vi "Import Data Sharing Framework with UDP Component.vi"() -> (3 "Output System Definition File":path)   [LabVIEW 2020, in "Data Sharing Framework Scripting Examples.lvlib"]
uses:
  Data Sharing Framework Scripting Examples.lvlib
  NationalInstruments.VeriStand.SystemDefinitionAPI
  <vilib>/addons/VeriStand Custom Device Scripting APIs/Data Sharing Framework/Data Sharing Framework Custom Device Scripting.lvlib
panel:
  in  "Launch Data Viewer":bool=TRUE
  in  "Data Server Frequency":dbl(ring)=10.0 items=["0.5 Hz"=0.5, "1.0 Hz"=1.0, "2.0 Hz"=2.0, "2.5 Hz"=2.5, "4.0 Hz"=4.0, "5.0 Hz"=5.0, "8.0 Hz"=8.0, "10.0 Hz"=10.0, "12.5 Hz"=12.5, "20.0 Hz"=20.0, "25.0 Hz"=25.0, "40.0 Hz"=40.0, "50.0 Hz"=50.0, "100.0 Hz"=100.0]
  in  "Enable Data Server":bool=TRUE
  # "Overview: Demonstrates using the Data Sharing Framework scripting API to import a UDP plugin for data communication between VeriStand and LabVIEW. \n\nInstructions:\n1. Specify data server parameters. \n2. You may specify configuration and system definition files on the Block Diagram.\n3. Run this VI to import the DSF configuration, save the system definition.\n4. From VeriStand, run the system definition to send shared data.\n5. From LabVIEW, run the UDP - Receiver VI to read shared data."
  # "Configure Data Server for Validation"
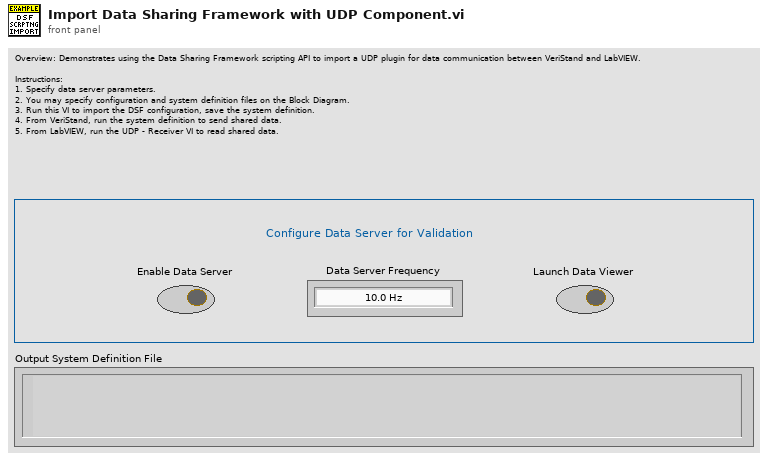
[diagram p1: front panel]
types:
  T1 = typedef "Custom Device API.lvlib/Custom Device Item Ref.ctl" = u64
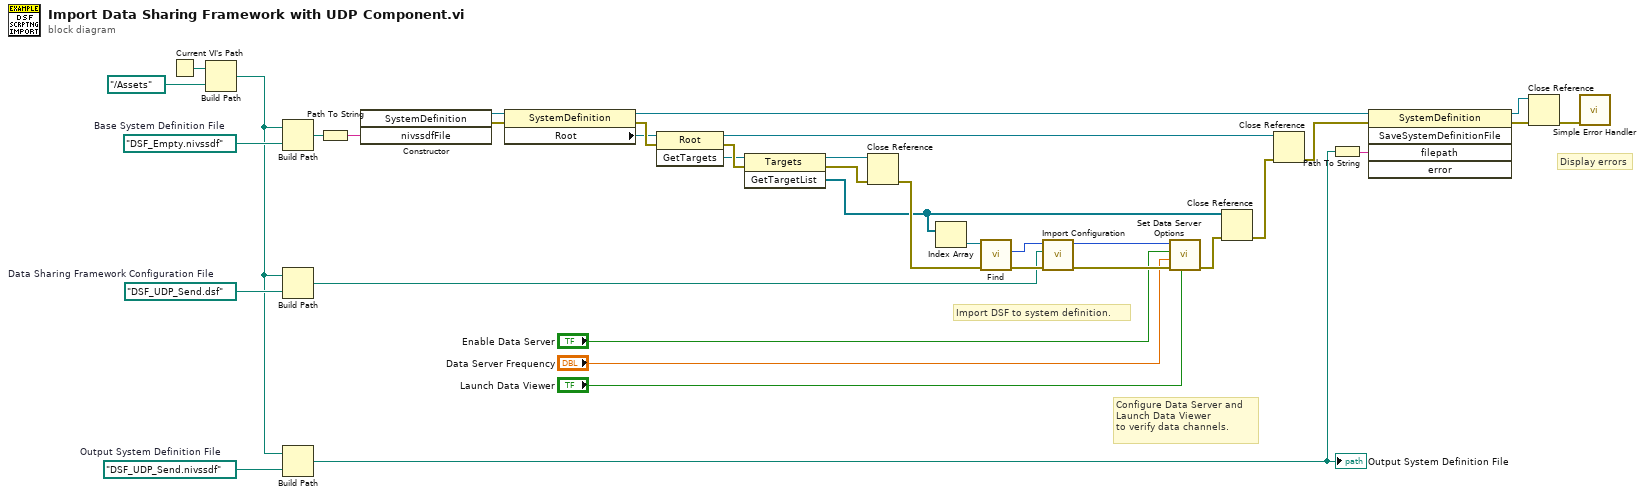
[diagram p0: block diagram]
diagram:
  w6 = path "DSF_Empty.nivssdf"  # Base System Definition File
  w2 = path "DSF_UDP_Send.nivssdf"  # Output System Definition File
  w5 = path "DSF_UDP_Send.dsf"  # Data Sharing Framework Configuration File
  # "Display errors"
  # "Import DSF to system definition."
  # "Configure Data Server and \nLaunch Data Viewer \nto verify data channels."
  n1 = Current VI's Path() -> (path=w9:path)
  n2 = Build Path(base path=w9, name or relative path=path "../Assets" ("relative path to assets")) -> (appended path=w3:path)
  n3 = Build Path(base path=w3, name or relative path=w6) -> (appended path=w7:path)
  n4 = Build Path(base path=w3, name or relative path=w5) -> (appended path=w4:path)
  n5 = Build Path(base path=w3, name or relative path=w2) -> (appended path=w1:path)
  "Output System Definition File" <- w1
  n6 = Path To String(path=w7) -> (string=w29:string)
  n7 = constructor class="SystemDefinition"("nivssdfFile"=w29) -> (reference out=w31:refnum<k24>, error out=w30:errorcluster)  [unwired: 3 in, 2 out]
  n8 = property class="SystemDefinition"(reference=w31, error in=w30) -> (reference out=w25:refnum<k24>, error out=w37:errorcluster, "Root"=w32:refnum<k24>)
  n9 = invoke class="Root" method="GetTargets"(reference=w32, error in=w37) -> (reference out=w27:refnum<k24>, error out=w36:errorcluster, "GetTargets"=w33:refnum<k24>)  [unwired: 1 in]
  n10 = invoke class="Targets" method="GetTargetList"(reference=w33, error in=w36) -> (reference out=w35:refnum<k24>, error out=w34:errorcluster, "GetTargetList"=w10:refnum<k24>[])  [unwired: 1 in]
  n11 = Close Reference(reference=w35, error in (no error)=w34) -> (error out=w14:errorcluster)
  n12 = Index Array(array=w10) -> (element=w12:refnum<k24>)  [unwired: 1 in]
  n13 = call <vilib>:"Find.vi"("error in"=w14, "target in"=w12) -> ("error out"=w13:errorcluster, "data sharing framework custom device"=w11:T1)  [unwired: 6 in, 2 out]
  n14 = call <vilib>:"Import Configuration.vi"("error in"=w13, "configuration file path"=w4, "data sharing framework custom device"=w11) -> ("error out"=w19:errorcluster, "data sharing framework custom device"=w20:T1)  [unwired: 7 in]
  n15 = call <vilib>:"Set Data Server Options.vi"("launch data viewer"="Launch Data Viewer", "error in"=w19, "data server frequency (Hz)"="Data Server Frequency", "enable data server"="Enable Data Server", "data sharing framework custom device in"=w20) -> ("error out"=w18:errorcluster)  [unwired: 4 in, 2 out]
  n16 = Close Reference(reference=w10, error in (no error)=w18) -> (error out=w28:errorcluster)
  n17 = Close Reference(reference=w27, error in (no error)=w28) -> (error out=w21:errorcluster)
  n18 = Path To String(path=w1) -> (string=w26:string)
  n19 = invoke class="SystemDefinition" method="SaveSystemDefinitionFile"(reference=w25, error in=w21, "filepath"=w26) -> (reference out=w23:refnum<k24>, error out=w24:errorcluster)  [unwired: 2 in, 3 out]
  n20 = Close Reference(reference=w23, error in (no error)=w24) -> (error out=w22:errorcluster)
  n21 = call <vilib>:"Simple Error Handler.vi"("error in (no error)"=w22) -> ()  [unwired: 1 in, 8 out]
